vi "set_phase_duration.vi"(8 "error in (no error)":errorcluster, 10 "phase duration":dbl[unit], 11 "IntrinsicImagingMG091001 in":refnum<class "DataCollectionMG091001IntrinsicImaging.lvclass">) -> (0 "error out":errorcluster, 3 "IntrinsicImagingMG091001 out":refnum<class "DataCollectionMG091001IntrinsicImaging.lvclass">)   [LabVIEW 2010, in "DataCollectionMG091001IntrinsicImaging.lvclass"]
uses:
  DataCollectionMG091001IntrinsicImaging.lvclass
  DataCollectionMG091001IntrinsicImaging.lvclass/DataCollectionMG091001IntrinsicImaging.ctl
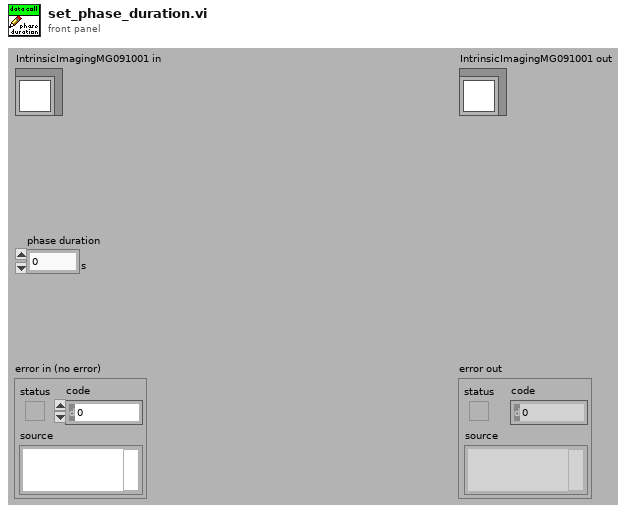
[diagram p1: front panel]
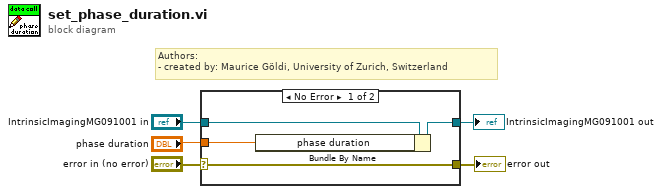
[diagram p0: block diagram]
diagram:
  # "Authors: \n- created by: Maurice Göldi, University of Zurich, Switzerland"
  n1 = case shown="No Error" "error in (no error)" {
    selector: "error in (no error)" -> [w9 w11]
    tunnel: [w9 w11] -> w4
    tunnel: [w6 w10] -> w2
    tunnel: "IntrinsicImagingMG091001 in" -> [w7 w10]
    tunnel: "phase duration" -> [w8 _]
    frame No Error {
      n2 = Bundle By Name(cluster=w7, "phase duration"=w8) -> (w6:refnum<class "DataCollectionMG091001IntrinsicImaging.lvclass">)
    }
    frame Error {
    }
  }
  "error out" <- w4
  "IntrinsicImagingMG091001 out" <- w2
